vi "Update_.vi"(0 "Pump_1AI_1DO_2DI in":refnum<class "NeedleValve.lvclass">, 11 "error in (no error)":errorcluster) -> (4 "Pump_1AI_1DO_2DI out":refnum<class "NeedleValve.lvclass">, 15 "error out":errorcluster)   [LabVIEW 2019, in "NeedleValve.lvclass"]
uses:
  NeedleValve.lvclass
  NeedleValve.lvclass/NeedleValve.ctl
  TypeDef/Needle Valve State.ctl
  modbus engine custom/MB_ENGINE_class/cmd enum.ctl
  modbus engine custom/MB_ENGINE_class/MB_ENGINE.lvclass
panel:
  out "Numeric":i32
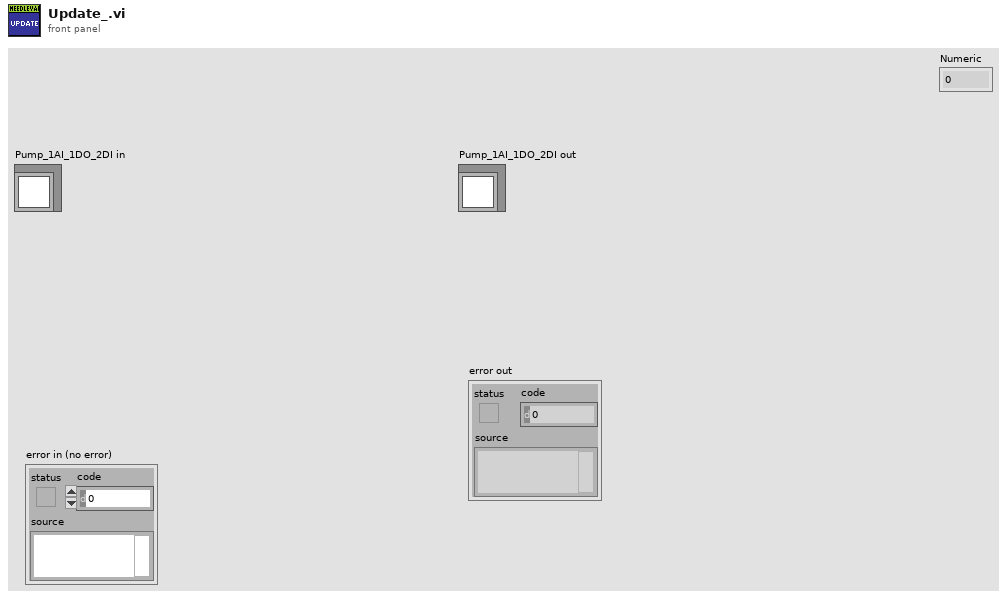
[diagram p1: front panel]
types:
  T1 = typedef "Needle Valve State.ctl" = enum16{"IDLE", "OPENING", "CLOSING", "STOP"}
  T2 = typedef "MB_ENGINE.lvclass/cmd enum.ctl" = u16
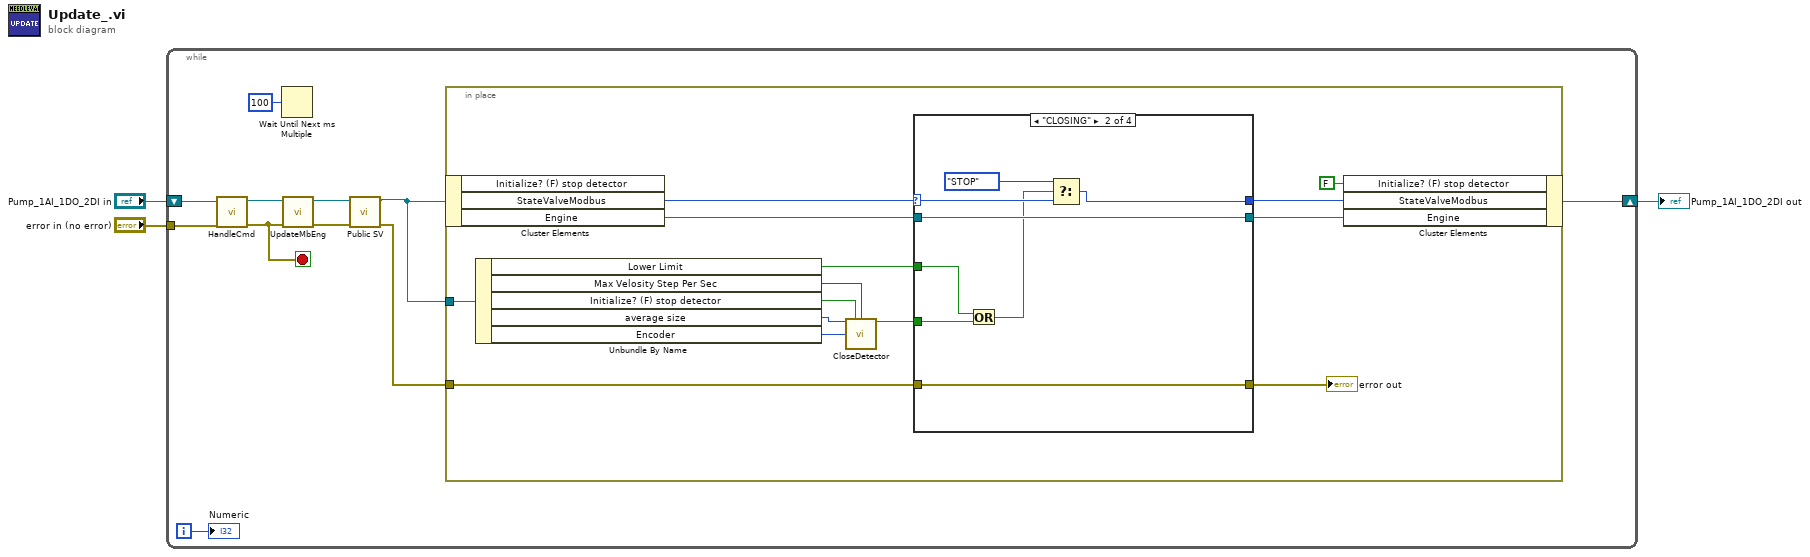
[diagram p0: block diagram]
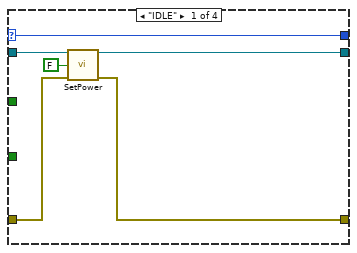
[diagram p2: hidden frame]
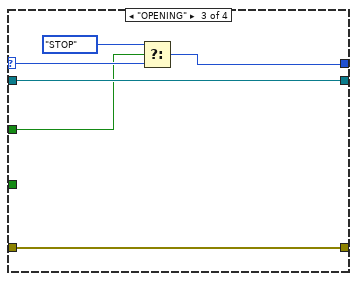
[diagram p3: hidden frame]
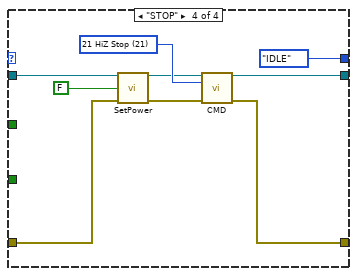
[diagram p4: hidden frame]
diagram:
  n1 = while {
    shift-right: [w11] -> w1
    shift-left: "Pump_1AI_1DO_2DI in" -> [w14]
    tunnel: "error in (no error)" -> [w13]
    i -> [w5]
    stop <- w4 stop-if-true
    n2 = call "HandleCmd.vi"("error in (no error)"=w13, "NeedleValve in"=w14) -> ("error out"=w4:errorcluster, "NeedleValve out"=w12:refnum<class "NeedleValve.lvclass">)  [unwired: 8 in]
    n3 = Wait Until Next ms Multiple(millisecond multiple=u32 100) -> ()  [unwired: 1 out]
    n4 = call "UpdateMbEng.vi"("error in (no error)"=w4, "NeedleValve in"=w12) -> ("error out"=w9:errorcluster, "NeedleValve out"=w10:refnum<class "NeedleValve.lvclass">)  [unwired: 8 in]
    n5 = call "Public SV.vi"("error in (no error)"=w9, "NeedleValve in"=w10) -> ("error out"=w8:errorcluster, "NeedleValve out"=w7:refnum<class "NeedleValve.lvclass">)  [unwired: 8 in]
    n6 = in-place {
      in-place-border: w8 -> [w23]
      in-place-border: w7 -> [w22]
      n7 = in-place-cluster #1(w7) -> ("StateValveModbus"=w28:T1, "Engine"=w25:refnum<class "MB_ENGINE.lvclass">)  [unwired: 1 out]
      n8 = Unbundle By Name(w22) -> ("Lower Limit"=w15:bool, "Max Velosity Step Per Sec"=w26:u16, "Initialize? (F) stop detector"=w20:bool, "average size"=w21:i32, "Encoder"=w19:i32)
      n9 = call "CloseDetector.vi"("Averaging Size"=w21, "Initialize? (F)"=w20, "MaxVelosity"=w26, "ENCODER"=w19) -> ("stop"=w18:bool)  [unwired: 11 in]
      n10 = case shown="\"CLOSING\"" w28 {
        selector: w28 -> [w34 w42 w48 _]
        tunnel: [w34 w41 w46 Needle_Valve_State."IDLE" ("StateValveModbus")] -> w27
        tunnel: w25 -> [w32 w39 w45 w52]
        tunnel: [w31 w39 w45 w51] -> w24
        tunnel: w23 -> [w30 w35 w44 w50]
        tunnel: w18 -> [_ w38 _ _]
        tunnel: [w29 w35 w44 w49] -> w16
        tunnel: w15 -> [_ w36 w43 _]
        frame "IDLE" {
          n11 = call "SetPower.vi"("class data in"=w32, "On"=FALSE, "error in (no error)"=w30) -> ("class data out"=w31:refnum<class "MB_ENGINE.lvclass">, "error out"=w29:errorcluster)  [unwired: 11 in]
        }
        frame "CLOSING" {
          n12 = Or(x=w36, y=w38) -> (x .or. y?=w37:bool)
          n13 = Select(t=Needle_Valve_State."STOP", s=w37, f=w42) -> (s? t:f=w41:T1)
        }
        frame "OPENING" {
          n14 = Select(t=Needle_Valve_State."STOP", s=w43, f=w48) -> (s? t:f=w46:T1)
        }
        frame "STOP" {
          w57 = T2 21 items=["0 Idle"=0, "1 GoTo Absolute Position"=1, "2 GoTo Relative"=2, "10 GoTo Home Position"=10, "11 Set Home Position"=11, "12 Set FindHome Mode"=12, "13 Reset FindHome Mode"=13, "14 Get FindHome State"=14, "20 Hard Stop"=20, "21 HiZ Stop"=21, "22 Soft Stop"=22, "30 Clear Fault"=30, "40 Encoder Set Home"=40, "70 Driver Init"=70] ("cmd to write")
          n15 = call "SetPower.vi"("class data in"=w52, "On"=FALSE, "error in (no error)"=w50) -> ("class data out"=w53:refnum<class "MB_ENGINE.lvclass">, "error out"=w54:errorcluster)  [unwired: 11 in]
          n16 = call "CMD.vi"("class data in"=w53, "cmd to write"=w57, "error in (no error)"=w54) -> ("class data out"=w51:refnum<class "MB_ENGINE.lvclass">, "error out"=w49:errorcluster)  [unwired: 11 in]
        }
      }
      "error out" <- w16
      n17 = in-place-cluster #1("Initialize? (F) stop detector"=FALSE, "StateValveModbus"=w27, "Engine"=w24) -> (w11:refnum<class "NeedleValve.lvclass">)
    }
    "Numeric" <- w5
  }
  "Pump_1AI_1DO_2DI out" <- w1
